vi "EquipmentServer.vi"() -> ()   [LabVIEW 2011]
doc: "LabServer6.vi receives the client settings via TCP and adjusts the instruments via PXI according to the client settings. Then it gets the result via PXI from the instruments and sends the result back to the client. It is composed of two parts: first, a loop that listens for each client to connect and adds them into a queue; and second, a loop that get client from the queue adjust the instruments and sends the result back."
uses:
  Server_Globals.vi
  Instance           9 23Saved   EquipmentServer .vi
panel:
  in  "Forced res. DMM":dbl
  in  "empty 2":refnum<k5>[](array[refnum])
  out "Reset":bool
  out "n:o measuerements":i32
  out "Client connected":bool
  in  "listen halted":bool
  in  "stop":bool
  in  "empty":refnum<k5>[](array[refnum])
  in  "Server port":u16=5001
  # "Disconnects all clients\nand shuts down server"
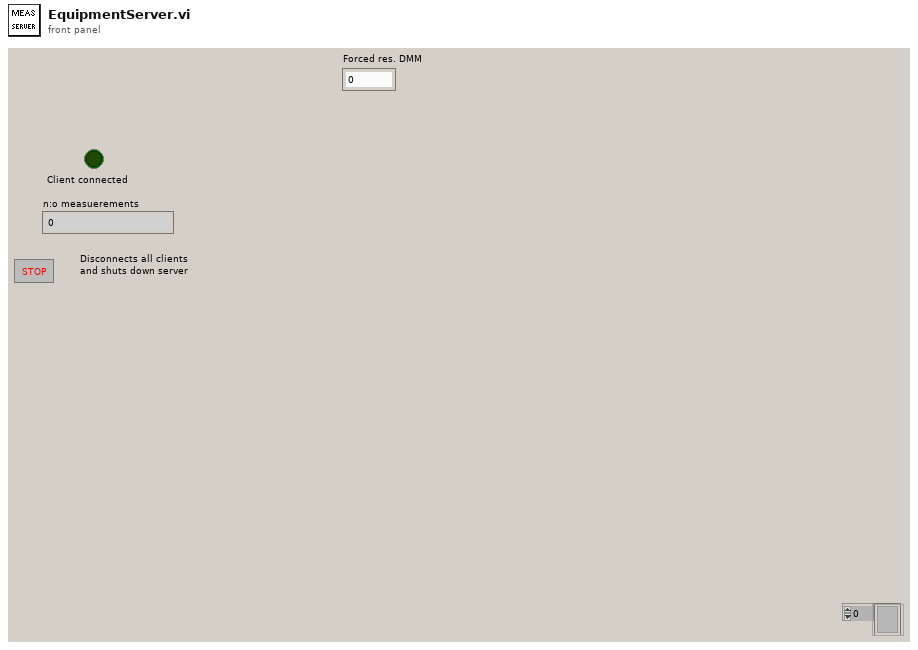
[diagram p1: front panel]
types:
  T1 = enum16{"GetElement", "AddElement", "Qlength", "ElementsInQueue"}
  T2 = cluster{"Global":cluster{"Port":i32, "Reset Time":i32, "Maximum Delay":i32}, "Instrument Adress":cluster{"5402":string, "4110":string, "5112":string, "USB":string, "4072":string}, "Log":cluster{"Log Level":u32, "Log File":path}, "Digital Multimeter":cluster{"0":string, "1":string, "2":string, "3":string, "4":string}, "Function Generator":cluster{"0":string, "1":string, "2":string, "3":string, "4":string}, "Digital Osciliscope":cluster{"0":string, "1":string, "2":string, "3":string, "4":string}, "DC Power Supply":cluster{"0":string, "1":string, "2":string, "3":string, "4":string}, "USB Interface":cluster{"0":string, "1":string, "2":string, "3":string, "4":string}, "Components":cluster{"Components type":string, "Components list":string}, "Matrix version":string, "Digital Multimeter Card 2":cluster{"0":string, "1":string, "2":string, "3":string, "4":string}}
  T3 = cluster{"Global":cluster{"Port":i32, "Reset Time":i32, "Maximum Delay":i32}, "Instrument Adress":cluster{"FGEN":string, "DC Power":string, "OSC":string, "USB":string, "DMM":string}, "Log":cluster{"Log Level":u32, "Log File":path}, "Digital Multimeter":cluster{"0":string, "1":string, "2":string, "3":string, "4":string}, "Function Generator":cluster{"0":string, "1":string, "2":string, "3":string, "4":string}, "Digital Osciliscope":cluster{"0":string, "1":string, "2":string, "3":string, "4":string}, "DC Power Supply":cluster{"0":string, "1":string, "2":string, "3":string, "4":string}, "USB Interface":cluster{"0":string, "1":string, "2":string, "3":string, "4":string}, "Components type":cluster{"Components type":string, "Components list":string}, "Matrix version":string, "Digital Multimeter Card 2":cluster{"0":string, "1":string, "2":string, "3":string, "4":string}}
  T4 = cluster{"0":string, "1":string, "2":string, "3":string, "4":string}
  T5 = cluster{"[0]":refnum<k15>, "[1]":refnum<k15>, "[2]":refnum<k15>, "[3]":refnum<k15>, "[4]":refnum<k15>}
  T6 = cluster{"[0]":refnum<visa-resource-name>, "[1]":refnum<visa-resource-name>, "[2]":refnum<visa-resource-name>, "[3]":refnum<visa-resource-name>, "[4]":refnum<visa-resource-name>}
  T7 = cluster{"I/O Settings":u64[], "Instrument Handle":cluster{"5402":refnum<k15>, " 5112":refnum<k15>, "4072":refnum<k15>, "USB":refnum<visa-resource-name>, "4110":refnum<k15>}, "Logfile":refnum<file>, "Log Level":i8, "Clear":i32[], "OS Set":cluster{"instrument handle out":refnum<k15>, "remaining string":string, "Settings":cluster{"Horizontal Conf.":cluster{"Min. Sample rate":dbl, "Reference position":dbl, "Record Length":i16}, "Channel A":cluster{"Enable":bool, "Vertical coupling":dbl, "Vertical range":dbl, "Vertical offset":dbl, "Probe attenuation":dbl}, "Channel B":cluster{"Enable":bool, "Vertical coupling":dbl, "Vertical range":dbl, "Vertical offset":dbl, "Probe attenuation":dbl}, "Trigger":cluster{"Source":enum8{"channel 1", "channel 2", "Imediate", "External trigger"}, "Slope":enum8{"Positive", "Negative"}, "Coupling":enum8{"AC", "DC"}, "Level":dbl, "Holdoff":dbl, "Delay":dbl, " Timeout":dbl, " Mode":enum8{"Normal", "Auto", "Auto Level"}}, "Measurements":cluster{"Measurement 1, Channel":enum8{"Channel 1", "Channel 2", "Channel 3", "Channel 4"}, "Measurement 1, Selection":u16, "Measurement 2, Channel":enum8{"Channel 1", "Channel 2", "Channel 3", "Channel 4"}, "Measurement 2,  Selection":u16, "Measurement 3, Channel":enum8{"Channel 1", "Channel 2", "Channel 3", "Channel 4"}, "Measurement 3, Selection 3":u16}}}, "DC Power Supply":cluster{"0":refnum<k15>, "1":refnum<k15>, "2":refnum<k15>, "3":refnum<k15>, "4":refnum<k15>}, "USB Interface":cluster{"0":refnum<visa-resource-name>, "1":refnum<visa-resource-name>, "2":refnum<visa-resource-name>, "3":refnum<visa-resource-name>, "4":refnum<visa-resource-name>}, "Function Generator":cluster{"0":refnum<k15>, "1":refnum<k15>, "2":refnum<k15>, "3":refnum<k15>, "4":refnum<k15>}, "Digital Multimeter":cluster{"0":refnum<k15>, "1":refnum<k15>, "2":refnum<k15>, "3":refnum<k15>, "4":refnum<k15>}, "Digital Osciliscope":cluster{"0":refnum<k15>, "1":refnum<k15>, "2":refnum<k15>, "3":refnum<k15>, "4":refnum<k15>}, "To M Server":string, "Adres":string[][], "Matrix version":string, "MD5":string, "Digital Multimeter Card 2":cluster{"0":string, "1":string, "2":string, "3":string, "4":string}}
  T8 = cluster{"0":refnum<k15>, "1":refnum<k15>, "2":refnum<k15>, "3":refnum<k15>, "4":refnum<k15>}
  T9 = cluster{"0":refnum<visa-resource-name>, "1":refnum<visa-resource-name>, "2":refnum<visa-resource-name>, "3":refnum<visa-resource-name>, "4":refnum<visa-resource-name>}
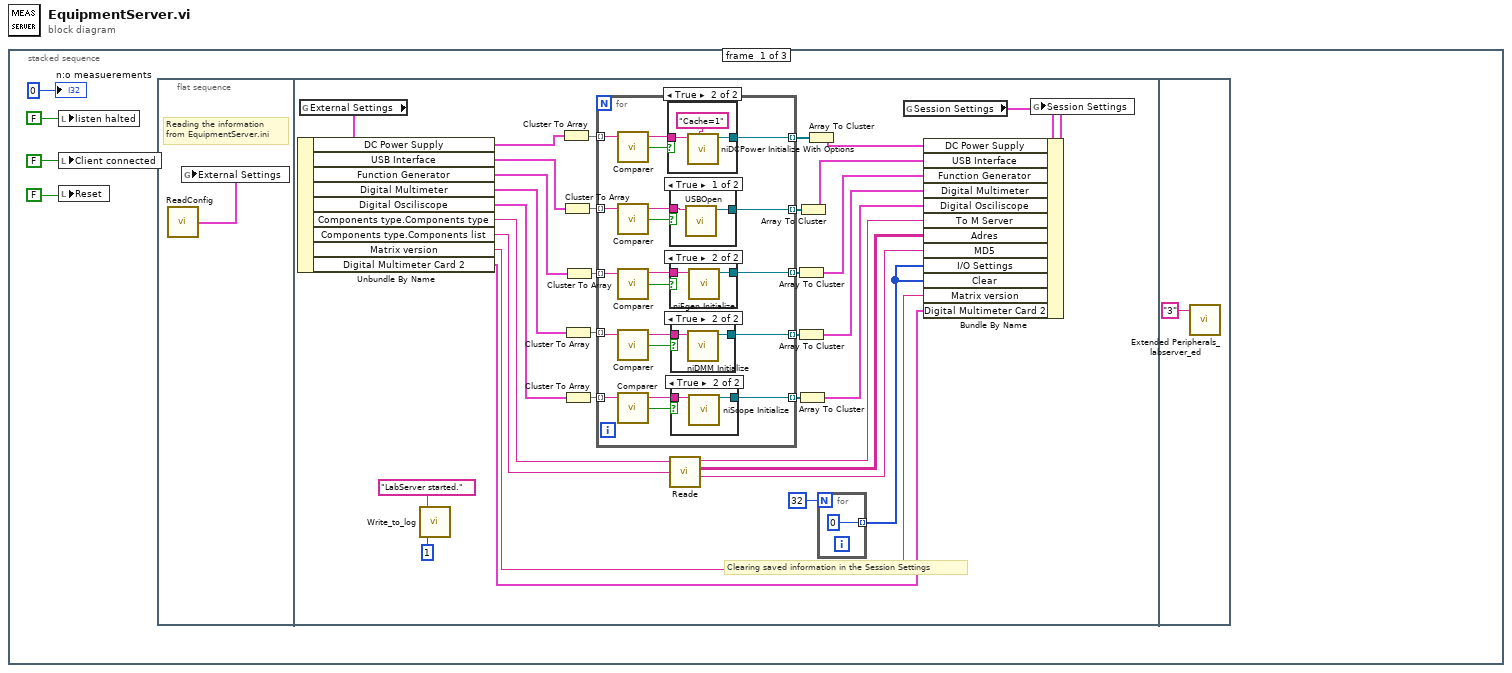
[diagram p0: block diagram]
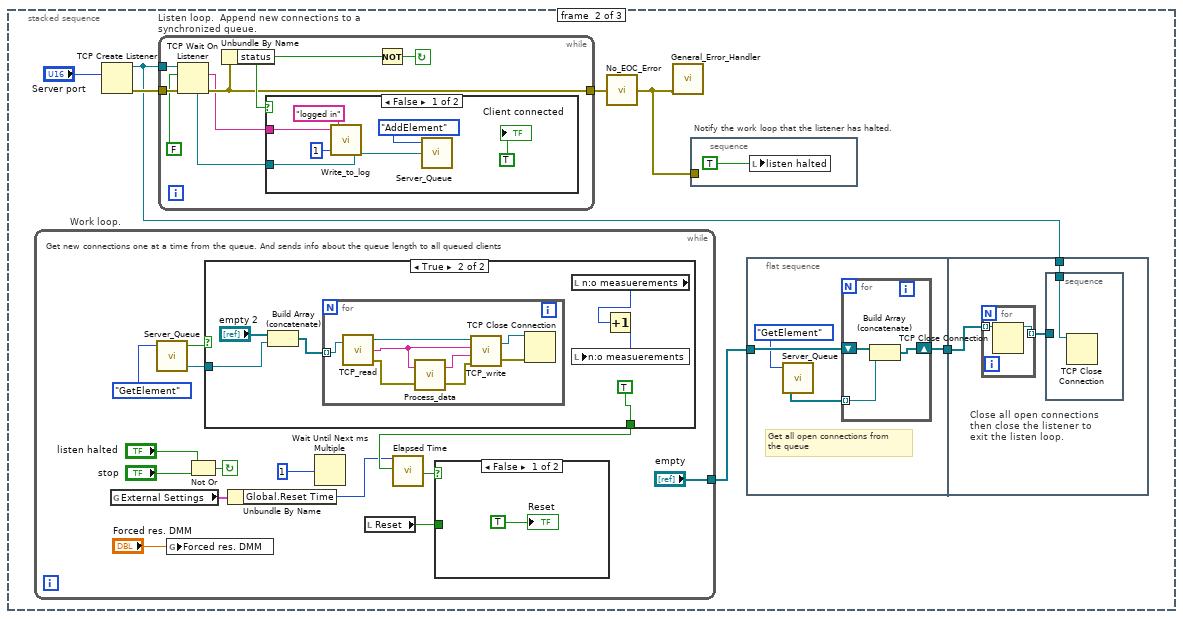
[diagram p7: hidden frame]
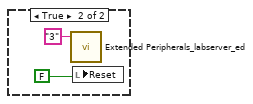
[diagram p9: hidden frame]
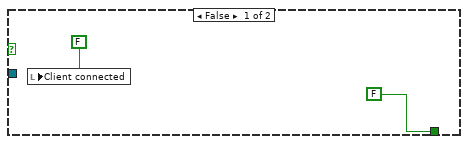
[diagram p10: hidden frame]
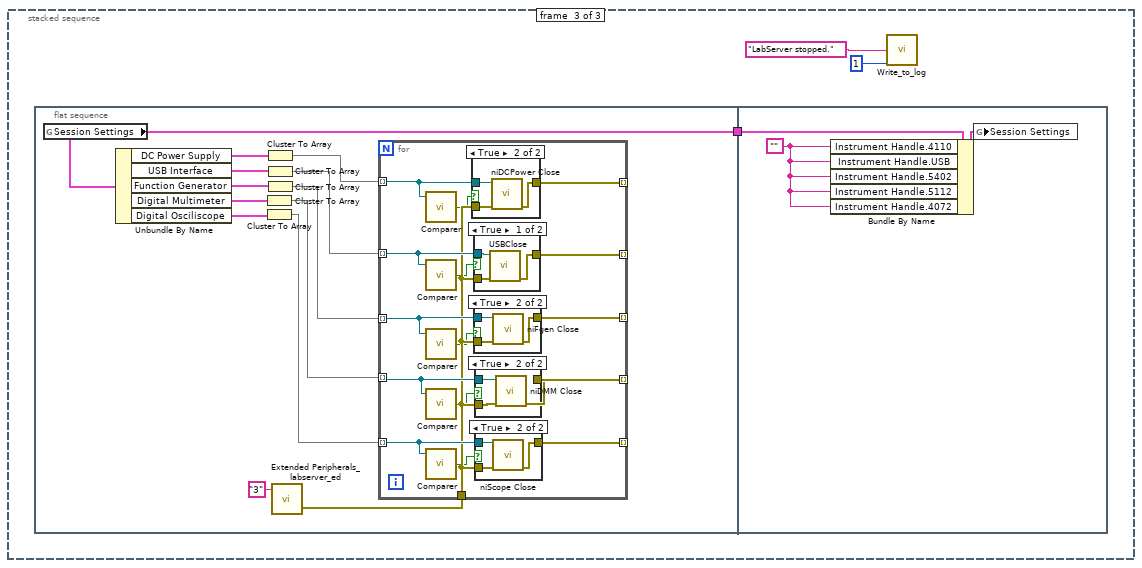
[diagram p12: hidden frame]
diagram:
  n1 = stacked-sequence {
    frame #0 {
      n2 = local write "listen halted"(FALSE) -> ()
      n3 = local write "Client connected"(FALSE) -> ()
      n4 = local write "Reset"(FALSE) -> ()
      n5 = flat-sequence {
        frame #0 {
          # "Reading the information\nfrom EquipmentServer.ini"
          n6 = call "ReadConfig.vi"() -> ("External Settings"=w5:T2)  [unwired: 2 in]
          n7 = global write "Server_Globals.vi" "External Settings"(w5) -> ()
        }
        frame #1 {
          # "Clearing saved information in the Session Settings"
          n8 = global read "Server_Globals.vi" "External Settings"() -> (w37:T3)
          n9 = Unbundle By Name(w37) -> ("DC Power Supply"=w33:T4, "USB Interface"=w30:T4, "Function Generator"=w25:T4, "Digital Multimeter"=w20:T4, "Digital Osciliscope"=w17:T4, "Components type.Components type"=w13:string, "Components type.Components list"=w9:string, "Matrix version"=w8:string, "Digital Multimeter Card 2"=w6:T4)
          n10 = call "Write_to_log.vi"("Type"=i8 1, "Message"="LabServer started.") -> ()  [unwired: 2 in]
          n11 = Cluster To Array(cluster=w33) -> (array=w32:string[])
          n12 = Cluster To Array(cluster=w30) -> (array=w31:string[])
          n13 = Cluster To Array(cluster=w20) -> (array=w21:string[])
          n14 = Cluster To Array(cluster=w17) -> (array=w16:string[])
          n15 = Cluster To Array(cluster=w25) -> (array=w24:string[])
          n16 = for {
            tunnel: w32 -> [w53] mode=indexing
            tunnel: [w59] -> w29 mode=indexing
            tunnel: w31 -> [w54] mode=indexing
            tunnel: [w56] -> w27 mode=indexing
            tunnel: w24 -> [w52] mode=indexing
            tunnel: [w57] -> w23 mode=indexing
            tunnel: w21 -> [w51] mode=indexing
            tunnel: [w58] -> w19 mode=indexing
            tunnel: w16 -> [w50] mode=indexing
            tunnel: [w55] -> w15 mode=indexing
            n17 = call "Comparer.vi"("Resource name"=w53) -> ("Boolean"=w45:bool, "Resource name"=w40:string)  [unwired: 3 in]
            n18 = call "Comparer.vi"("Resource name"=w54) -> ("Boolean"=w46:bool, "Resource name"=w41:string)  [unwired: 3 in]
            n19 = call "Comparer.vi"("Resource name"=w52) -> ("Boolean"=w47:bool, "Resource name"=w42:string)  [unwired: 3 in]
            n20 = call "Comparer.vi"("Resource name"=w51) -> ("Boolean"=w48:bool, "Resource name"=w44:string)  [unwired: 3 in]
            n21 = call "Comparer.vi"("Resource name"=w50) -> ("Boolean"=w49:bool, "Resource name"=w43:string)  [unwired: 3 in]
            n22 = case shown="True" w45 {
              tunnel: [w69 w71] -> w59
              tunnel: w40 -> [w69 w70]
              frame False {
              }
              frame True {
                n23 = call <instrlib>:"niDCPower Initialize With Options.vi"("option string"="Cache=1", "resource name"=w70) -> ("instrument handle out"=w71:refnum<k15>)  [unwired: 8 in, 1 out]
              }
            }
            n24 = case shown="True" w46 {
              tunnel: [w74 w75] -> w56
              tunnel: w41 -> [w73 w75]
              frame True {
                n25 = call "USBOpen.vi"("USB"=w73) -> ("VISA Resource Name"=w74:refnum<visa-resource-name>)  [unwired: 9 in, 1 out]
              }
              frame False {
              }
            }
            n26 = case shown="True" w47 {
              tunnel: w42 -> [w66 w68]
              tunnel: [w66 w67] -> w57
              frame False {
              }
              frame True {
                n27 = call <instrlib>:"niFgen Initialize.vi"("Resource Name"=w68) -> ("Instrument Handle Out"=w67:refnum<k15>)  [unwired: 9 in, 1 out]
              }
            }
            n28 = case shown="True" w48 {
              tunnel: w44 -> [w63 w65]
              tunnel: [w63 w64] -> w58
              frame False {
              }
              frame True {
                n29 = call <instrlib>:"niDMM Initialize.vi"("Instrument Descriptor"=w65) -> ("instrument handle out"=w64:refnum<k15>)  [unwired: 9 in, 1 out]
              }
            }
            n30 = case shown="True" w49 {
              tunnel: w43 -> [w60 w62]
              tunnel: [w60 w61] -> w55
              frame False {
              }
              frame True {
                n31 = call <instrlib>:"niScope Initialize.vi"("resource name"=w62) -> ("instrument handle"=w61:refnum<k15>)  [unwired: 13 in, 1 out]
              }
            }
          }
          n32 = call "Reade.vi"("Components type"=w13, "ComponentsList"=w9) -> ("To M Server"=w12:string, "Address"=w11:string[][], "MD5"=w7:string)  [unwired: 1 in, 1 out]
          n33 = Array To Cluster(array=w23) -> (cluster=w22:T5)
          n34 = Array To Cluster(array=w19) -> (cluster=w18:T5)
          n35 = Array To Cluster(array=w15) -> (cluster=w14:T5)
          n36 = Array To Cluster(array=w27) -> (cluster=w26:T6)
          n37 = Array To Cluster(array=w29) -> (cluster=w28:T5)
          n38 = for {
            N: 32 -> [_]
            tunnel: [0] -> w10 mode=indexing
          }
          n39 = global read "Server_Globals.vi" "Session Settings"() -> (w35:T7)
          n40 = Bundle By Name(cluster=w35, "DC Power Supply"=w28, "USB Interface"=w26, "Function Generator"=w22, "Digital Multimeter"=w18, "Digital Osciliscope"=w14, "To M Server"=w12, "Adres"=w11, "MD5"=w7, "I/O Settings"=w10, "Clear"=w10, "Matrix version"=w8, "Digital Multimeter Card 2"=w6) -> (w36:T7)
          n41 = global write "Server_Globals.vi" "Session Settings"(w36) -> ()
        }
        frame #2 {
          n42 = call "Extended Peripherals_labserver_ed.vi"("Command In"="3") -> ()  [unwired: 2 in, 2 out]
        }
      }
      "n:o measuerements" <- 0
    }
    frame #1 {
      # "Notify the work loop that the listener has halted."
      n43 = while "Work loop." {
        tunnel: ["empty"] -> w82
        stop <- w111 continue-if-true
        # "Get new connections one at a time from the queue. And sends info about the queue length to all queued clients"
        n44 = global read "Server_Globals.vi" "External Settings"() -> (w100:T3)
        n45 = call "Server_Queue.vi"("Mode"=T1."GetElement") -> ("value"=w107:refnum<k5>, "valid?"=w108:bool)  [unwired: 1 in, 2 out]
        n46 = global write "DMM_Res" "Forced res. DMM"("Forced res. DMM") -> ()
        n47 = Not Or(1:"stop", 2:"listen halted") -> (0:w111:bool)
        n48 = case shown="True" w108 {
          tunnel: w107 -> [_ w119]
          tunnel: [FALSE TRUE] -> w103
          frame False {
            n49 = local write "Client connected"(FALSE) -> ()
          }
          frame True {
            n50 = Build Array (concatenate)("empty 2", w119) -> (w118:refnum<k5>[])
            n51 = for {
              tunnel: w118 -> [w131] mode=indexing
              n52 = call "TCP_read.vi"("Client ID In"=w131) -> ("Client ID out"=w130:refnum<k5>, "Dataout"=w124:string, "error out (no error)"=w129:errorcluster)  [unwired: 1 in]
              n53 = call "Process_data.vi"("error in (no error)"=w129, "String to process"=w124) -> ("error out (no error)"=w128:errorcluster, "String to send"=w127:string)
              n54 = call "TCP_write.vi"("error in (no error)"=w128, "Data to send"=w127, "Parameter to Server"=w124, "TCP ID in"=w130) -> ("error out (no error)"=w126:errorcluster, "TCP ID out"=w125:refnum<k5>)
              n55 = TCP Close Connection(connection ID=w125, error in (no error)=w126) -> ()  [unwired: 1 in, 2 out]
            }
            n56 = local read "n:o measuerements"() -> (w122:i32)
            n57 = Increment(x=w122) -> (x+1=w121:i32)
            n58 = local write "n:o measuerements"(w121) -> ()
          }
        }
        n59 = Unbundle By Name(w100) -> ("Global.Reset Time"=w99:i32)
        n60 = Wait Until Next ms Multiple(millisecond multiple=u32 1) -> ()  [unwired: 1 out]
        n61 = local read "Reset"() -> (w101:bool)
        n62 = call "Elapsed Time"("Time Target (s)"=w99, "Reset"=w103) -> ("Time has Elapsed"=w102:bool)  [unwired: 10 in, 7 out]
        n63 = case shown="False" w102 {
          tunnel: w101 -> [_ w113]
          frame False {
            "Reset" <- TRUE
          }
          frame True {
            n64 = case shown="False" w113 {
              frame False {
              }
              frame True {
                n65 = call "Extended Peripherals_labserver_ed.vi"("Command In"="3") -> ()  [unwired: 2 in, 2 out]
                n66 = local write "Reset"(FALSE) -> ()
              }
            }
          }
        }
      }
      n67 = TCP Create Listener(10:"Server port") -> (0:w83:errorcluster, 3:w78:refnum<k5>)  [unwired: 4 in, 1 out]
      n68 = while "Listen loop.  Append new connections to a synchronized queue." {
        tunnel: w78 -> [w137]
        tunnel: w83 -> [w138]
        tunnel: [w133] -> w80
        stop <- w139 continue-if-true
        n69 = TCP Wait On Listener(8:w138, 10:FALSE, 11:w137) -> (0:w133:errorcluster, 2:w132:string, 4:w135:refnum<k5>)  [unwired: 1 in, 2 out]
        n70 = Unbundle By Name(w133) -> ("status"=w136:bool)
        n71 = case shown="False" w136 {
          tunnel: w135 -> [w140 _]
          tunnel: w132 -> [w141 _]
          frame False {
            n72 = call "Write_to_log.vi"("TCP Refnum"=w140, "Type"=i8 1, "Message"="logged in", "Cient ip"=w141) -> ()
            n73 = call "Server_Queue.vi"("new value"=w140, "Mode"=T1."AddElement") -> ()  [unwired: 4 out]
            "Client connected" <- TRUE
          }
          frame True {
          }
        }
        n74 = Not(x=w136) -> (.not. x?=w139:bool)
      }
      n75 = call "No_EOC_Error.vi"("error in"=w80) -> ("error out"=w81:errorcluster)  [unwired: 4 in]
      n76 = call "General_Error_Handler.vi"("error in (no error)"=w81) -> ()  [unwired: 10 in, 5 out]
      n77 = stacked-sequence {
        tunnel: w81 -> [_]
        frame #0 {
          n78 = local write "listen halted"(TRUE) -> ()
        }
      }
      n79 = flat-sequence {
        tunnel: w82 -> [w88]
        tunnel: [w87] -> w79
        tunnel: w79 -> [w92]
        tunnel: w78 -> [w93]
        frame #0 {
          # "Get all open connections from \nthe queue"
          n80 = call "Server_Queue.vi"("Mode"=T1."GetElement") -> ("Elements in Queue"=w86:refnum<k5>[])  [unwired: 1 in, 3 out]
          n81 = for {
            shift-right: [w90] -> w87
            shift-left: w88 -> [w91]
            tunnel: w86 -> [w89] mode=indexing
            n82 = Build Array (concatenate)(w91, w89) -> (w90:refnum<k5>[])
          }
        }
        frame #1 {
          # "Close all open connections then close the listener to exit the listen loop."
          n83 = for {
            tunnel: [w96] -> w94 mode=indexing
            tunnel: w92 -> [w95] mode=indexing
            n84 = TCP Close Connection(connection ID=w95) -> (connection ID out=w96:refnum<k5>)  [unwired: 2 in, 1 out]
          }
          n85 = stacked-sequence {
            tunnel: w93 -> [w97]
            tunnel: w94 -> [_]
            frame #0 {
              n86 = TCP Close Connection(connection ID=w97) -> ()  [unwired: 2 in, 2 out]
            }
          }
        }
      }
    }
    frame #2 {
      n87 = flat-sequence {
        tunnel: [w161] -> w147
        tunnel: w147 -> [w200]
        frame #0 {
          n88 = global read "Server_Globals.vi" "Session Settings"() -> (w161:T7)
          n89 = Unbundle By Name(w161) -> ("DC Power Supply"=w160:T8, "USB Interface"=w158:T9, "Function Generator"=w156:T8, "Digital Multimeter"=w154:T8, "Digital Osciliscope"=w152:T8)
          n90 = Cluster To Array(cluster=w154) -> (array=w153:refnum<k15>[])
          n91 = Cluster To Array(cluster=w152) -> (array=w151:refnum<k15>[])
          n92 = Cluster To Array(cluster=w160) -> (array=w159:refnum<k15>[])
          n93 = Cluster To Array(cluster=w158) -> (array=w157:refnum<visa-resource-name>[])
          n94 = Cluster To Array(cluster=w156) -> (array=w155:refnum<k15>[])
          n95 = call "Extended Peripherals_labserver_ed.vi"("Command In"="3") -> ("error out (no error)"=w150:errorcluster)  [unwired: 2 in, 1 out]
          n96 = for {
            tunnel: w159 -> [w172] mode=indexing
            tunnel: [w178] -> _ mode=indexing
            tunnel: w157 -> [w173] mode=indexing
            tunnel: [w175] -> _ mode=indexing
            tunnel: w155 -> [w171] mode=indexing
            tunnel: [w176] -> _ mode=indexing
            tunnel: w153 -> [w170] mode=indexing
            tunnel: [w177] -> _ mode=indexing
            tunnel: w151 -> [w169] mode=indexing
            tunnel: [w174] -> _ mode=indexing
            tunnel: w150 -> [w168]
            n97 = call "Comparer.vi"("Resource name"=w172) -> ("Boolean"=w163:bool)  [unwired: 3 in, 1 out]
            n98 = call "Comparer.vi"("Resource name"=w173) -> ("Boolean"=w164:bool)  [unwired: 3 in, 1 out]
            n99 = call "Comparer.vi"("Resource name"=w171) -> ("Boolean"=w165:bool)  [unwired: 3 in, 1 out]
            n100 = call "Comparer.vi"("Resource name"=w170) -> ("Boolean"=w166:bool)  [unwired: 3 in, 1 out]
            n101 = call "Comparer.vi"("Resource name"=w169) -> ("Boolean"=w167:bool)  [unwired: 3 in, 1 out]
            n102 = case shown="True" w163 {
              tunnel: [w191 w194] -> w178
              tunnel: w172 -> [_ w193]
              tunnel: w168 -> [w191 w192]
              frame False {
              }
              frame True {
                n103 = call <instrlib>:"niDCPower Close.vi"("error in (no error)"=w192, "instrument handle"=w193) -> ("error out"=w194:errorcluster)  [unwired: 9 in]
              }
            }
            n104 = case shown="True" w164 {
              tunnel: [w197 w198] -> w175
              tunnel: w173 -> [w196 _]
              tunnel: w168 -> [w195 w198]
              frame True {
                n105 = call "USBClose.vi"("error in (no error)"=w195, "USB"=w196) -> ("error out"=w197:errorcluster)  [unwired: 9 in]
              }
              frame False {
              }
            }
            n106 = case shown="True" w165 {
              tunnel: w171 -> [_ w190]
              tunnel: [w187 w189] -> w176
              tunnel: w168 -> [w187 w188]
              frame False {
              }
              frame True {
                n107 = call <instrlib>:"niFgen Close.vi"("error in (no error)"=w188, "Instrument Handle"=w190) -> ("error out"=w189:errorcluster)  [unwired: 9 in]
              }
            }
            n108 = case shown="True" w166 {
              tunnel: w170 -> [_ w186]
              tunnel: [w183 w185] -> w177
              tunnel: w168 -> [w183 w184]
              frame False {
              }
              frame True {
                n109 = call <instrlib>:"niDMM Close.vi"("error in (no error)"=w184, "instrument handle"=w186) -> ("error out"=w185:errorcluster)  [unwired: 9 in]
              }
            }
            n110 = case shown="True" w167 {
              tunnel: w169 -> [_ w182]
              tunnel: [w179 w181] -> w174
              tunnel: w168 -> [w179 w180]
              frame False {
              }
              frame True {
                n111 = call <instrlib>:"niScope Close.vi"("instrument handle"=w182, "error in"=w180) -> ("error out"=w181:errorcluster)  [unwired: 13 in]
              }
            }
          }
        }
        frame #1 {
          w199 = ""
          n112 = Bundle By Name(cluster=w200, "Instrument Handle.4110"=w199, "Instrument Handle.USB"=w199, "Instrument Handle.5402"=w199, "Instrument Handle.5112"=w199, "Instrument Handle.4072"=w199) -> (w201:T7)
          n113 = global write "Server_Globals.vi" "Session Settings"(w201) -> ()
        }
      }
      n114 = call "Write_to_log.vi"("Type"=i8 1, "Message"="LabServer stopped.") -> ()  [unwired: 2 in]
    }
  }
